vi "Empty Host Software Package.vi"() -> (0 "Software Package":T1)   [LabVIEW 2021, in "Acquisition.lvlib"]
doc: "(inline VI) Return an empty Host Software Package. Use in-place of a block diagram constant.\n\nA cluster of strings representing the unique package ID and version of a software package installed on the running Host system."
uses:
  Acquisition.lvlib
  Host Software Package.ctl
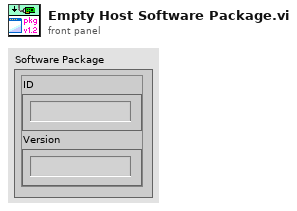
[diagram p1: front panel]
types:
  T1 = typedef "Acquisition.lvlib/Host Software Package.ctl" = cluster{"ID":string, "Version":string}
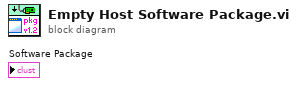
[diagram p0: block diagram]
diagram:
